vi "filtrowanie z rosbaga współrzędnych geograficznych.vi"() -> ()   [LabVIEW 2012]
doc: "Zadaniem pliku testowego jest odfiltrowanie długości i szerokości geograficzne z rosbaga i zapisanie ich do pliku tekstowego, który wykorzystywany jest w pliku tekstowym odczyt współrzędnych z GPS"
uses:
  <vilib>/Utility/file.llb/Write To Spreadsheet File (DBL).vi
  <vilib>/regexp/Match Regular Expression.xnode
panel:
  in  "file path (dialog if empty) 2":path
  out "Array":dbl[][](array[numeric]) format="%.8f"
  in  "file path (dialog if empty)":path=path "C:/Moje dane/Politechnika Łódzka/Semestr VII/Praca inżynierska/Moduł map + robot/mapy i współrzędne/wspolrzedne.txt"
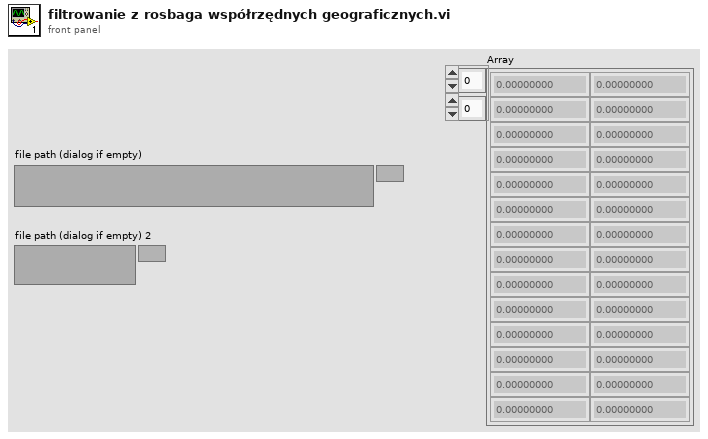
[diagram p1: front panel]
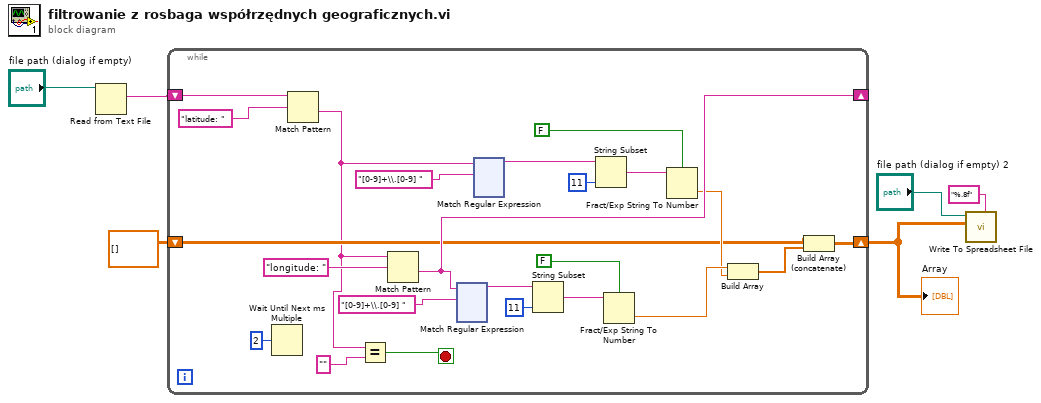
[diagram p0: block diagram]
diagram:
  n1 = Read from Text File(file (use dialog)="file path (dialog if empty)") -> (text=w5:string)  [unwired: 3 in, 3 out]
  n2 = while {
    shift-right: [w16] -> _
    shift-left: w5 -> [w17]
    shift-right: [w12] -> w3
    shift-left: dbl[][] [] -> [w11]
    stop <- w7 stop-if-true
    n3 = Wait Until Next ms Multiple(millisecond multiple=u32 2) -> ()  [unwired: 1 out]
    n4 = Match Pattern(string=w17, regular expression="latitude: ") -> (after substring=w9:string)  [unwired: 1 in, 3 out]
    n5 = Equal?(x=w9, y="") -> (x = y?=w7:bool)
    n6 = Match Pattern(string=w9, regular expression="longitude: ") -> (after substring=w16:string)  [unwired: 1 in, 3 out]
    n7 = xnode "Match Regular Expression"("input string"=w16, "regular expression"="[0-9]+\\.[0-9] ") -> ("before match"=w22:string)  [unwired: 4 in, 4 out]
    n8 = xnode "Match Regular Expression"("input string"=w9, "regular expression"="[0-9]+\\.[0-9] ") -> ("before match"=w25:string)  [unwired: 4 in, 4 out]
    n9 = String Subset(string=w22, length (rest)=11 ("length (rest)")) -> (substring=w21:string)  [unwired: 1 in]
    n10 = String Subset(string=w25, length (rest)=11 ("length (rest)")) -> (substring=w26:string)  [unwired: 1 in]
    n11 = Fract/Exp String To Number(use system decimal point (T)=FALSE, string=w21) -> (number=w15:dbl)  [unwired: 2 in, 1 out]
    n12 = Fract/Exp String To Number(use system decimal point (T)=FALSE, string=w26) -> (number=w14:dbl)  [unwired: 2 in, 1 out]
    n13 = Build Array(w15, w14) -> (w13:dbl[])
    n14 = Build Array (concatenate)(w11, w13) -> (w12:dbl[][])
  }
  "Array" <- w3
  n15 = call-poly <vilib>:"Write To Spreadsheet File.vi"("format (%.3f)"="%.8f", "2D data"=w3, "file path (dialog if empty)"="file path (dialog if empty) 2") -> ()  [unwired: 5 in, 1 out]
